vi "PeaksInPlot.vi"(0 "Format String":string, 1 "Unit String":string, 2 "X-Axis Array":dbl[][](array[numeric]) format="%.2f", 3 "Data Array":dbl[][](array[numeric]) format="%.2f", 4 "Cursor Plot":u32) -> (5 "Peaks: X":dbl[](array[numeric]) format="%.3f", 6 "Peak Position Strings []":string[](array[string]), 7 "Peaks: Y":dbl[](array[numeric]) format="%.3e")   [LabVIEW 2025]
doc: "Author: Scott Hannahs <sth@magnet.fsu.edu>\n\nThis software is licensed for use under the “MIT License\"\nCopyright (c) 2025 Scott Hannahs, sth@sth@magnet.sthnet.net\n\nPermission is hereby granted, free of charge, to any person obtaining a copy of this software and associated documentation files (the \"Software\"), to deal in the Software without restriction, including without limitation the rights to use, copy, modify, merge, publish, distribute, sublicense, and/or sell copies of the Software, and to permit persons to whom the Software is furnished to do so, subject to the following conditions: The above copyright notice and this permission notice shall be included in all copies or substantial portions of the Software.\n\nTHE SOFTWARE IS PROVIDED \"AS IS\", WITHOUT WARRANTY OF ANY KIND, EXPRESS OR IMPLIED, INCLUDING BUT NOT LIMITED TO THE WARRANTIES OF MERCHANTABILITY, FITNESS FOR A PARTICULAR PURPOSE AND NONINFRINGEMENT. IN NO EVENT SHALL THE AUTHORS OR COPYRIGHT HOLDERS BE LIABLE FOR ANY CLAIM, DAMAGES OR OTHER LIABILITY, WHETHER IN AN ACTION OF CONTRACT, TORT OR OTHERWISE, ARISING FROM, OUT OF OR IN CONNECTION WITH THE SOFTWARE OR THE USE OR OTHER DEALINGS IN THE SOFTWARE."
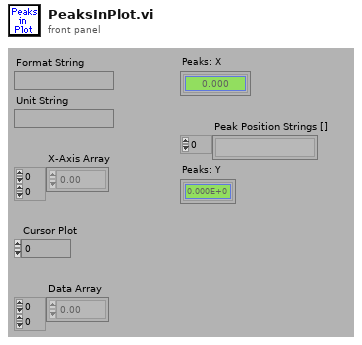
[diagram p1: front panel]
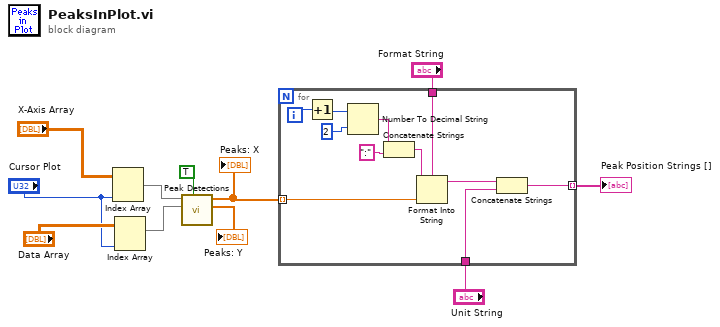
[diagram p0: block diagram]
diagram:
  n1 = Index Array(array="X-Axis Array", index (col)="Cursor Plot") -> (element=w4:dbl[])  [unwired: 1 in]
  n2 = Index Array(array="Data Array", index (col)="Cursor Plot") -> (element=w5:dbl[])  [unwired: 1 in]
  n3 = call "Peak Detections.vi"("View Result?"=TRUE, "Input y data"=w5, "Input x data"=w4) -> ("Peak Amplitudes"=→"Peaks: Y":dbl[], "Peak Locations"=w8:dbl[])  [unwired: 2 in, 5 out]
  "Peaks: X" <- w8
  n4 = for {
    tunnel: w8 -> [w22] mode=indexing
    tunnel: "Format String" -> [w17]
    tunnel: [w14] -> w9 mode=indexing
    tunnel: "Unit String" -> [w15]
    i -> [w12]
    n5 = Increment(x=w12) -> (x+1=w13:i32)
    n6 = Number To Decimal String(number=w13, width (-)=i16 2) -> (decimal integer string=w20:string)
    n7 = Concatenate Strings(w20, ":") -> (w18:string)
    n8 = Format Into String(format string=w17, initial string=w18, w22) -> (resulting string=w16:string)  [unwired: 1 in, 1 out]
    n9 = Concatenate Strings(w16, w15) -> (w14:string)
  }
  "Peak Position Strings []" <- w9
